vi "Divide I32 By 2.vi"(11 "Value":i32) -> (3 "Value/2":i32)   [LabVIEW 2021, in "Math.lvlib"]
uses:
  Math.lvlib
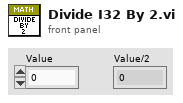
[diagram p1: front panel]
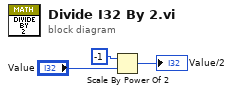
[diagram p0: block diagram]
diagram:
  n1 = Scale By Power Of 2(n=i16 -1, x="Value") -> (x*2^n=→"Value/2":i32)
